vi "Configure Signaling RF Subcarrier Spacing.vi"(8 "error in (no error)":errorcluster, 9 "Subcarrier Spacing (0)":i32, 10 "Cell Name (\"Cell Name\")":string="Cell Name", 11 "VISA resource name":refnum<visa-resource-name>) -> (0 "error out":errorcluster, 3 "VISA resource name out":refnum<visa-resource-name>)   [LabVIEW 2020, in "Rohde&Schwarz CMWXP NR FR1 Measurement.lvlib"]
doc: "Selects the subcarrier spacing.\n\nAttribute:\nRSCMWXPNRFR1M_ATTR_SIGNALING_RF_SUBCARRIER_SPACING\n\nRemote-control command:\n[CONFigure:]SIGNaling:NRADio:CELL:RFSettings:SSPacing"
uses:
  <instrlib>/Rohde&Schwarz CMWXP NR FR1 Measurement/Rohde&Schwarz CMWXP NR FR1 Measurement.lvlib
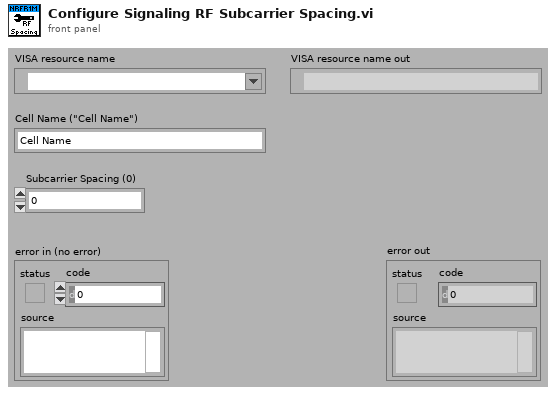
[diagram p1: front panel]
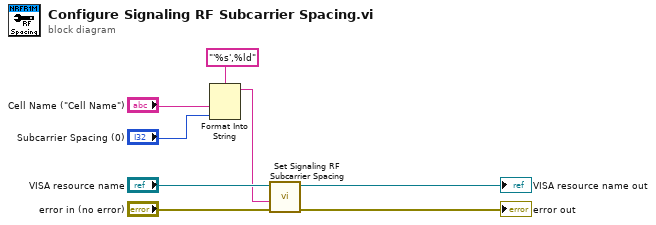
[diagram p0: block diagram]
diagram:
  n1 = Format Into String(format string="'%s',%ld", "Cell Name (\"Cell Name\")", "Subcarrier Spacing (0)") -> (resulting string=w1:string)  [unwired: 2 in, 1 out]
  n2 = call "Set Signaling RF Subcarrier Spacing"("error in (no error)"="error in (no error)", "Signaling RF Subcarrier Spacing ()"=w1, "instrument handle"="VISA resource name") -> ("error out"=→"error out":errorcluster, "instrument handle out"=→"VISA resource name out":refnum<visa-resource-name>)  [unwired: 7 in]
